vi "Start Points.vi"(8 "error in":errorcluster, 11 "Sample PI Control in":refnum<class "Sample PI Control.lvclass">) -> (0 "error out":errorcluster, 3 "Sample PI Control out":refnum<class "Sample PI Control.lvclass">)   [LabVIEW 2023, in "Sample PI Control.lvclass"]
uses:
  Sample PI Control.lvclass
  Sample PI Control.lvclass/Sample PI Control.ctl
  Task/Task Base/Task Base.lvclass
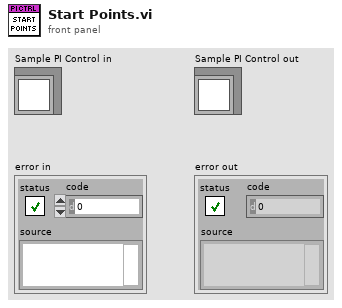
[diagram p1: front panel]
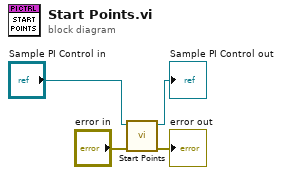
[diagram p0: block diagram]
diagram:
  n1 = call-parent "Start Points.vi"("error in"="error in", "Task Base in"="Sample PI Control in") -> ("error out"=→"error out":errorcluster, "Task Base out"=→"Sample PI Control out":refnum<class "Sample PI Control.lvclass">)  [unwired: 8 in]
